vi "Pre Launch Init.vi"(11 "MediatorBusMonitor in":refnum<class "MediatorBusMonitor.lvclass">) -> (0 "error out":errorcluster, 3 "MediatorBusMonitor out":refnum<class "MediatorBusMonitor.lvclass">)   [LabVIEW 2015, in "Mediator.lvlib" / "MediatorBusMonitor.lvclass"]
doc: "(<B>Filename</B>: Actor Framework.lvlib:Actor.lvclass:Pre Launch Init.vi)\n\nDefines behavior that occurs after the Launch Nested Actor method is invoked but before the actor's Actor Core method begins running.\n\nBy default, this method does nothing. A descendant class may override it to define behavior."
uses:
  MediatorBusMonitor.lvclass
  MediatorBusMonitor Messages/Update Front Panel Msg/Update Front Panel Msg.lvclass
  MediatorBusMonitor.lvclass/MediatorBusMonitor.ctl
  <vilib>/ActorFramework/Actor/Actor.lvclass/Actor.ctl
  <vilib>/ActorFramework/Message Enqueuer/Message Enqueuer.lvclass/Message Enqueuer.ctl
  <vilib>/ActorFramework/Message Enqueuer/Init from Existing Queue.vi
  IMediator/IMediatorBusMonitor/MediatorBusMonitor/IMediatorBusMonitor.lvclass
  <vilib>/ActorFramework/Message Enqueuer/Message Enqueuer.lvclass
  <vilib>/Composed Systems/Current Value Table/CurrentValueTable.lvclass
  <vilib>/ActorFramework/Actor/Actor.lvclass
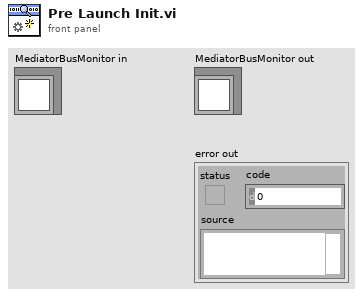
[diagram p1: front panel]
types:
  T1 = typedef "CurrentValueTable.lvlib/CurrentValueTable.lvclass/CurrentValueTable Reference.ctl" = refnum<data-value>
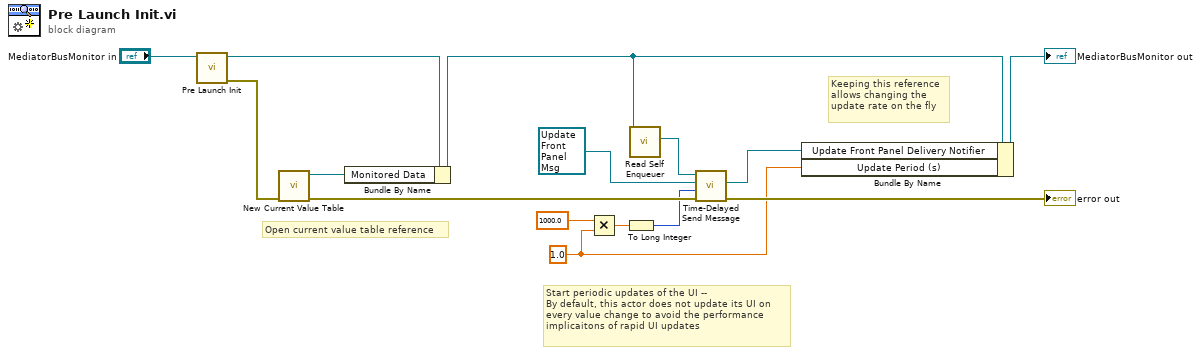
[diagram p0: block diagram]
diagram:
  w2 = 1.0 ("Milliseconds To Wait")
  # "Keeping this reference\nallows changing the\nupdate rate on the fly"
  # "Start periodic updates of the UI --\nBy default, this actor does not update its UI on\nevery value change to avoid the performance\nimplicaitons of rapid UI updates"
  # "Open current value table reference"
  n1 = call-parent "Pre Launch Init.vi"("IEventAggregator in"="MediatorBusMonitor in") -> ("error out"=w12:errorcluster, "IEventAggregator out"=w15:refnum<class "MediatorBusMonitor.lvclass">)  [unwired: 9 in]
  n2 = call <vilib>:"New Current Value Table.vi"("error in (no error)"=w12) -> ("error out"=w11:errorcluster, "Current Value Table"=w13:T1)  [unwired: 9 in]
  n3 = Bundle By Name(cluster=w15, "Monitored Data"=w13) -> (w8:refnum<class "MediatorBusMonitor.lvclass">)
  n4 = Multiply(x=1000.0, y=w2) -> (x*y=w4:dbl)
  n5 = To Long Integer(number=w4) -> (32bit integer=w1:i32)
  n6 = call <vilib>:"Read Self Enqueuer.vi"("Actor"=w8) -> ("Self Enqueuer"=w7:refnum<class "Message Enqueuer.lvclass">)  [unwired: 10 in]
  n7 = call <vilib>:"Time-Delayed Send Message.vi"("error in (no error)"=w11, "Milliseconds To Wait"=w1, "Message"=refnum<class "Update Front Panel Msg.lvclass"> refnum ("Mediator.lvlib:Update Front Panel Msg.lvclass"), "Message Enqueuer"=w7) -> ("error out"=→"error out":errorcluster, "Delivery Notifier"=w5:refnum<notifier>)  [unwired: 6 in]
  n8 = Bundle By Name(cluster=w8, "Update Front Panel Delivery Notifier"=w5, "Update Period (s)"=w2) -> (→"MediatorBusMonitor out":refnum<class "MediatorBusMonitor.lvclass">)
